vi "Create Selection.vi"(8 "error in (no error)":errorcluster, 10 "Shape":refnum<data-value>) -> (0 "error out":errorcluster, 3 "SelectedShape Reference":refnum<data-value>)   [LabVIEW 2017, in "LV Image Editor Framework.lvlib" / "Selection.lvclass"]
uses:
  Selection.lvclass
  Shape/Shape.lvclass
  C:/Github/LIEF/Forms/Shape/Shape.lvclass
  Shape/Shape.lvclass/Shape.ctl
  Selection.lvclass/Selection.ctl
  Shape/Read Bounds.vi
  Shape/Read Movable.vi
  Shape/Read Color.vi
  Shape/Read Selection Visible.vi
  Shape/Write Movable.vi
  Shape/Write Color.vi
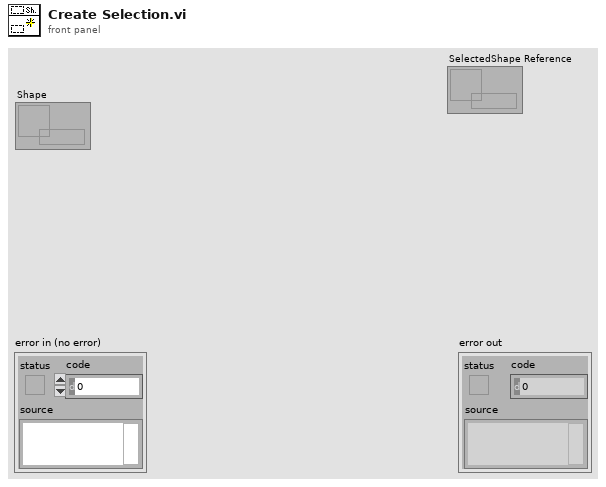
[diagram p1: front panel]
types:
  T1 = cluster{"Left":i32, "Top":i32, "Right":i32, "Bottom":i32}
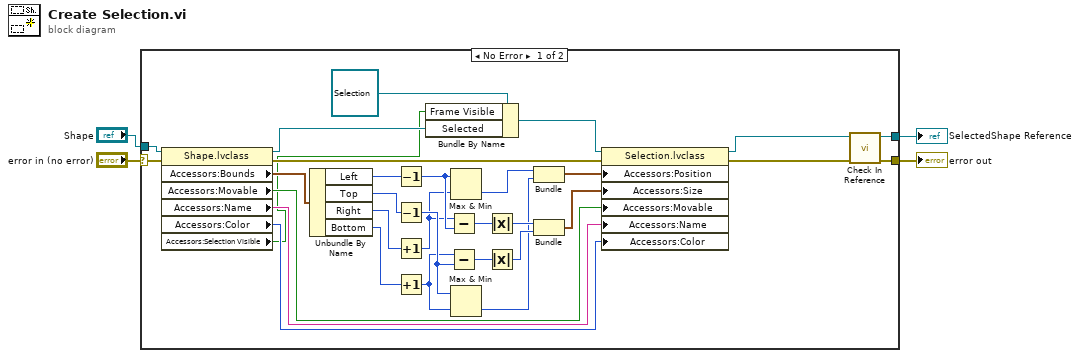
[diagram p0: block diagram]
diagram:
  n1 = case shown="No Error" "error in (no error)" {
    selector: "error in (no error)" -> [w24 w36]
    tunnel: [w26 w36] -> w3
    tunnel: [w25 _] -> w1
    tunnel: "Shape" -> [w29 _]
    frame No Error {
      n2 = property class="Shape.lvclass"(reference=w29, error in=w24) -> (reference out=w27:refnum<data-value>, error out=w12:errorcluster, "Accessors:Bounds"=w28:T1, "Accessors:Movable"=w15:bool, "Accessors:Name"=w14:string, "Accessors:Color"=w13:u32, "Accessors:Selection Visible"=w10:bool)
      n3 = Unbundle By Name(w28) -> ("Left"=w31:i32, "Top"=w30:i32, "Right"=w34:i32, "Bottom"=w35:i32)
      n4 = Decrement(x=w31) -> (x-1=w23:i32)
      n5 = Decrement(x=w30) -> (x-1=w22:i32)
      n6 = Increment(x=w34) -> (x+1=w16:i32)
      n7 = Increment(x=w35) -> (x+1=w21:i32)
      n8 = Bundle By Name(cluster=refnum<class "Selection.lvclass"> refnum ("Selection in"), "Frame Visible"=w10, "Selected"=w27) -> (w8:refnum<class "Selection.lvclass">)
      n9 = Subtract(x=w16, y=w23) -> (x-y=w33:i32)
      n10 = Subtract(x=w21, y=w22) -> (x-y=w32:i32)
      n11 = Max & Min(x=w23, y=w16) -> (min(x,y)=w18:i32)  [unwired: 1 out]
      n12 = Max & Min(x=w22, y=w21) -> (min(x,y)=w17:i32)  [unwired: 1 out]
      n13 = Absolute Value(x=w33) -> (abs(x)=w20:i32)
      n14 = Absolute Value(x=w32) -> (abs(x)=w19:i32)
      n15 = Bundle(w18, w17) -> (w6:cluster{i32, i32})  [unwired: 1 in]
      n16 = Bundle(w20, w19) -> (w5:cluster{i32, i32})  [unwired: 1 in]
      n17 = property class="Selection.lvclass"(reference=w8, error in=w12, "Accessors:Position"=w6, "Accessors:Size"=w5, "Accessors:Movable"=w15, "Accessors:Name"=w14, "Accessors:Color"=w13) -> (reference out=w7:refnum<class "Selection.lvclass">, error out=w11:errorcluster)
      n18 = call "Check In Reference.vi"("error in (no error)"=w11, "Shape in"=w7) -> ("error out"=w26:errorcluster, "Shape Reference"=w25:refnum<data-value>)  [unwired: 8 in]
    }
    frame Error {
    }
  }
  "error out" <- w3
  "SelectedShape Reference" <- w1
